vi "Create Source Sequence Parameters.vi"(10 "Reference values":T2={"dcpower session reservation"=refnum, "Source handle array"=[], "Source channel name array"=[], "Load handle"="", "Load channel name"="", "Source voltage values"=[], "Load current values"=[], "Number of steps"=0, "Source sequence name"="", "Source terminal name"="", "Measure terminal name"="", "scope session reservation"=refnum, "Scope handles"=[], "connection map"={}, "instrument info map array"=[], "Enable TClk"=FALSE, "dmm session reservation"=refnum, "dmm handle array"=[], "DMM Trigger Source"=enum."Immediate", "DMM Sample Trigger"=enum."TTL 0", "Measurement Results"={"Status"="", "Voltage values"=[], "Source sweep points"=0, "Load sweep points"=0, "Source voltages"=[], "Source currents"=[], "Load voltages"=[], "Load currents"=[], "Load voltage deviation"=[], "Efficiency"=[], "Maximum efficiency"=[], "Minimum load voltage"=[], "Maximum load voltage"=[], "Minimum load regulation"=[], "Maximum load regulation"=[], "waveform pins"=[], "waveform sites"=[], "waveform t0 array"=[], "waveform dt array"=[], "waveform length array"=[], "concatenated waveform Y"=[]}, "Additional measurements"={"voltage measurements from all sources"=[], "current measurements from all sources"=[], "all dmm measurements"=[], "all scope waverforms"=[]}}, 11 "measurement configuration":T10={"Mode of operation"=enum."Perform measurement", "DUT setup time"=1.0, "Source delay"=0.005, "Aperture time"=0.005, "Nominal output voltage"=3.3, "Source pin name array"=[], "Source pin name index for efficiency"=0, "Source sense array"=[], "Source current limit array"=[], "Source maximum power array"=[], "Source start voltage array"=[], "Source stop voltage array"=[], "Source voltage sweep points"=4, "Use Source voltage array"=FALSE, "Source voltage concatenated array"=[], "Source voltage array size"=[], "Load pin name"="", "Load sense"=1009, "Load voltage limit range"=6.0, "Load sweep type"="Logarithmic", "Load start current"=0.1, "Load stop current"=24.0, "Load current sweep points/points per decade"=10, "Use Load current array"=FALSE, "Load current array"=[], "Pin Names for Scope"=[], "vertical range"=[], "vertical offset"=[], "probe attenuation"=[], "vertical coupling"=[], "channel enabled"=[], "input impedance"=[], "max input frequency"=[], "min sample rate"=[], "reference position"=[], "min record length"=[], "enforce realtime"=[], "dmm pin names"=[], "dmm function array"=[], "dmm resolution in digits array"=[], "dmm range array"=[]} {"dmm function array" items=["DC Volts", "AC Volts", "DC Current", "AC Current", "2-wire Resistance", "4-wire Resistance", "Diode", "Frequency", "Period", "AC Volts DC Coupled", "Capacitance", "Inductance", "Temperature"]; "Source sense array" items=["Local"=1008, "Remote"=1009]; "dmm resolution in digits array" items=["3 1/2"=3.5, "4 1/2"=4.5, "5 1/2"=5.5, "6 1/2"=6.5, "7 1/2"=7.5]; "input impedance" items=["1 mega ohm"=0, "50 ohms"=2]; "vertical coupling" items=["AC", "DC", "Ground"]; "Load sense" items=["Local"=1008, "Remote"=1009]}) -> (3 "source sequence parameters":T1[](array[typedef]) {"Transient Response" items=["Slow"=1041, "Normal"=1038, "Fast"=1039, "Custom"=1042]; "Sense" items=["Local"=1008, "Remote"=1009]})   [LabVIEW 2021, in "Efficiency And Load Regulation with Pin Map.lvlib"]
uses:
  Efficiency And Load Regulation with Pin Map.lvlib
  Measurement Configuration.ctl
  <instrlib>/niScope/Controls/niScope vertical coupling.ctl
  <instrlib>/niDMM/nidmm.llb/niDMM Resolution in Digits.ctl
  Reference values.ctl
  <vilib>/Plug-In SDKs/Clients/Session Management V1/Session Reservation/Session Reservation.lvclass
  common/Instrument Control/Scope/TClk/Instrument Info.ctl
  common/Instrument Control/Scope Parameters.ctl
  <instrlib>/niDMM/nidmm.llb/niDMM Trigger.ctl
  <instrlib>/niDMM/nidmm.llb/niDMM Sample Trigger.ctl
  Measurement Results.ctl
  Additional measurements.ctl
  common/Instrument Control/DCPower Parameters for Adv Sequence.ctl
  common/PMIC Common.lvlib
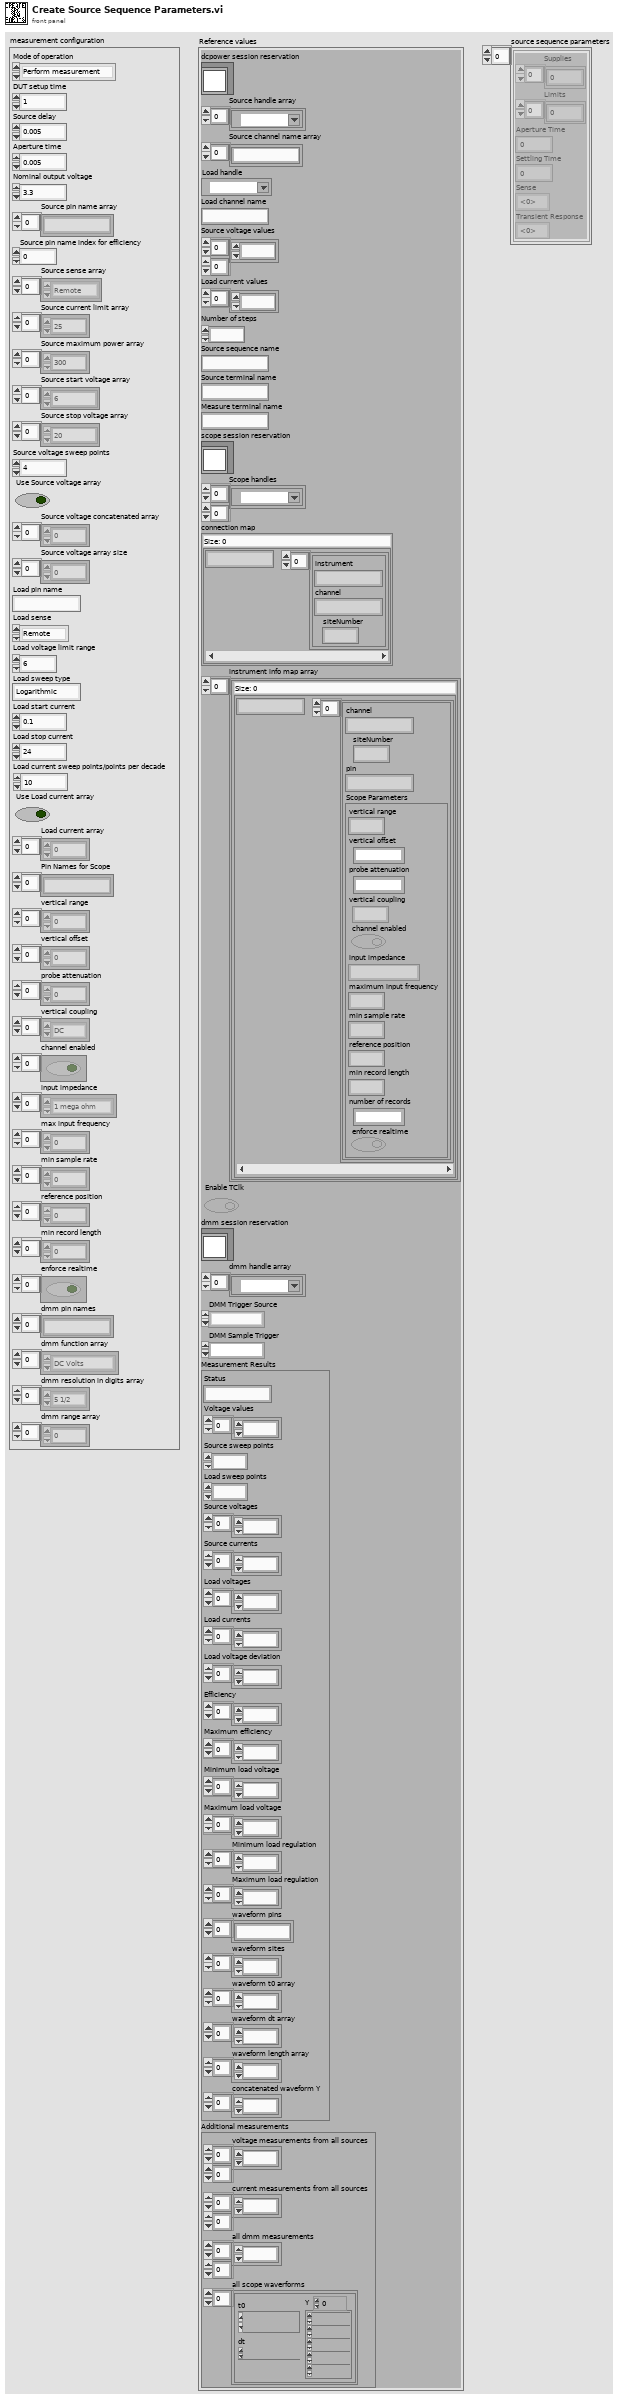
[diagram p1: front panel]
types:
  T1 = typedef "PMIC Common.lvlib/DCPower Parameters for Adv Sequence.ctl" = cluster{"Supplies":dbl[], "Limits":dbl[], "Aperture Time":dbl, "Settling Time":dbl, "Sense":i32, "Transient Response":i32}
  T2 = typedef "Efficiency And Load Regulation with Pin Map.lvlib/Reference values.ctl" = cluster{"dcpower session reservation":refnum<class "Session Reservation.lvclass">, "Source handle array":refnum<k15>[], "Source channel name array":string[], "Load handle":refnum<k15>, "Load channel name":string, "Source voltage values":dbl[][], "Load current values":dbl[], "Number of steps":i32, "Source sequence name":string, "Source terminal name":string, "Measure terminal name":string, "scope session reservation":refnum<class "Session Reservation.lvclass">, "Scope handles":refnum<k15>[][], "connection map":map{string, T3[]}, "instrument info map array":map{string, cluster{"channel":string, "siteNumber":i32, "pin":string, "Scope Parameters":T4}[]}[], "Enable TClk":bool, "dmm session reservation":refnum<class "Session Reservation.lvclass">, "dmm handle array":refnum<k15>[], "DMM Trigger Source":T6, "DMM Sample Trigger":T7, "Measurement Results":T8, "Additional measurements":T9}
  T3 = typedef "PMIC Common.lvlib/Instrument Info.ctl" = cluster{"instrument":string, "channel":string, "siteNumber":i32}
  T4 = typedef "PMIC Common.lvlib/Scope Parameters.ctl" = cluster{"vertical range":dbl, "vertical offset":dbl, "probe attenuation":dbl, "vertical coupling":T5, "channel enabled":bool, "input impedance":u32, "maximum input frequency":dbl, "min sample rate":dbl, "reference position":dbl, "min record length":i32, "number of records":i32, "enforce realtime":bool}
  T5 = typedef "niScope vertical coupling.ctl" = i32
  T6 = typedef "niDMM Trigger.ctl" = enum16{"Immediate", "External", "TTL 0", "TTL 1", "TTL 2", "TTL 3", "TTL 4", "TTL 5", "TTL 6", "Software", "TTL 7", "PXI Star", "LBR Trig 1", "Aux Trig 1"}
  T7 = typedef "niDMM Sample Trigger.ctl" = enum16{"Immediate", "External", "TTL 0", "TTL 1", "TTL 2", "TTL 3", "TTL 4", "TTL 5", "TTL 6", "Interval", "Software", "TTL 7", "PXI Star", "LBR Trig 1", "Aux Trig 1"}
  T8 = typedef "Efficiency And Load Regulation with Pin Map.lvlib/Measurement Results.ctl" = cluster{"Status":string, "Voltage values":dbl[], "Source sweep points":i32, "Load sweep points":i32, "Source voltages":dbl[], "Source currents":dbl[], "Load voltages":dbl[], "Load currents":dbl[], "Load voltage deviation":dbl[], "Efficiency":dbl[], "Maximum efficiency":dbl[], "Minimum load voltage":dbl[], "Maximum load voltage":dbl[], "Minimum load regulation":dbl[], "Maximum load regulation":dbl[], "waveform pins":string[], "waveform sites":i32[], "waveform t0 array":dbl[], "waveform dt array":dbl[], "waveform length array":i32[], "concatenated waveform Y":dbl[]}
  T9 = typedef "Efficiency And Load Regulation with Pin Map.lvlib/Additional measurements.ctl" = cluster{"voltage measurements from all sources":dbl[][], "current measurements from all sources":dbl[][], "all dmm measurements":dbl[][], "all scope waverforms":waveform(dbl)[]}
  T10 = typedef "Efficiency And Load Regulation with Pin Map.lvlib/Measurement Configuration.ctl" = cluster{"Mode of operation":enum32{"Power on the DUT", "Perform measurement", "Power off the DUT"}, "DUT setup time":dbl, "Source delay":dbl, "Aperture time":dbl, "Nominal output voltage":dbl, "Source pin name array":string[], "Source pin name index for efficiency":i32, "Source sense array":i32[], "Source current limit array":dbl[], "Source maximum power array":dbl[], "Source start voltage array":dbl[], "Source stop voltage array":dbl[], "Source voltage sweep points":i32, "Use Source voltage array":bool, "Source voltage concatenated array":dbl[], "Source voltage array size":i32[], "Load pin name":string, "Load sense":i32, "Load voltage limit range":dbl, "Load sweep type":string, "Load start current":dbl, "Load stop current":dbl, "Load current sweep points/points per decade":i32, "Use Load current array":bool, "Load current array":dbl[], "Pin Names for Scope":string[], "vertical range":dbl[], "vertical offset":dbl[], "probe attenuation":dbl[], "vertical coupling":T5[], "channel enabled":bool[], "input impedance":u32[], "max input frequency":dbl[], "min sample rate":dbl[], "reference position":dbl[], "min record length":i32[], "enforce realtime":bool[], "dmm pin names":string[], "dmm function array":u32[], "dmm resolution in digits array":T11[], "dmm range array":dbl[]}
  T11 = typedef "niDMM Resolution in Digits.ctl" = dbl
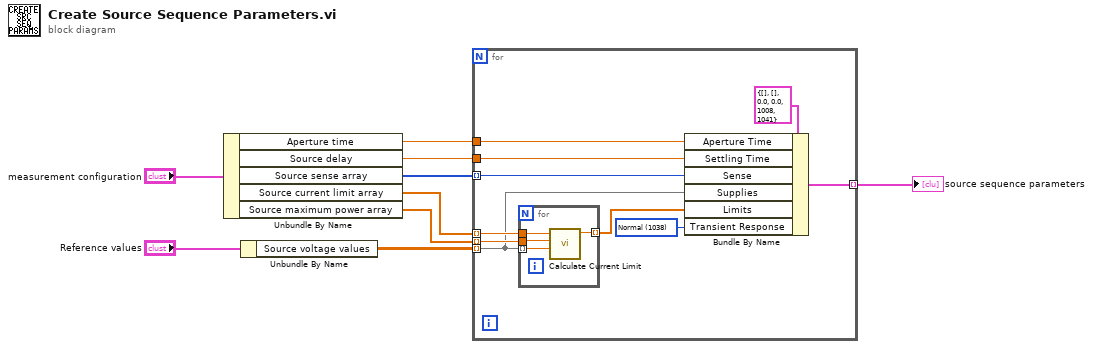
[diagram p0: block diagram]
diagram:
  n1 = Unbundle By Name("measurement configuration") -> ("Aperture time"=w9:dbl, "Source delay"=w8:dbl, "Source sense array"=w7:i32[], "Source current limit array"=w6:dbl[], "Source maximum power array"=w5:dbl[])
  n2 = Unbundle By Name("Reference values") -> ("Source voltage values"=w2:dbl[][])
  n3 = for {
    tunnel: w9 -> [w18]
    tunnel: w8 -> [w17]
    tunnel: w7 -> [w16] mode=indexing
    tunnel: w6 -> [w15] mode=indexing
    tunnel: w5 -> [w14] mode=indexing
    tunnel: w2 -> [w11] mode=indexing
    tunnel: [w10] -> w1 mode=indexing
    w12 = 1038 items=["Slow"=1041, "Normal"=1038, "Fast"=1039, "Custom"=1042] ("Transient Response")
    n4 = for {
      tunnel: w11 -> [w21] mode=indexing
      tunnel: w14 -> [w23]
      tunnel: w15 -> [w22]
      tunnel: [w20] -> w13 mode=indexing
      n5 = call "Calculate Current Limit.vi"("Voltage value"=w21, "Maximum power"=w23, "Current limit in"=w22) -> ("Current limit out"=w20:dbl)  [unwired: 8 in]
    }
    n6 = Bundle By Name(cluster=T1 {"Supplies"=[], "Limits"=[], "Aperture Time"=0.0, "Settling Time"=0.0, "Sense"=1008, "Transient Response"=1041} ("Parameters for Adv Sequence"), "Aperture Time"=w18, "Settling Time"=w17, "Sense"=w16, "Supplies"=w11, "Limits"=w13, "Transient Response"=w12) -> (w10:T1)
  }
  "source sequence parameters" <- w1
